vi "Unescape String.vi"(11 "string":string) -> (3 "parsed string":string)   [LabVIEW 2017, in "NI_LVConfig.lvlib"]
uses:
  <vilib>/Utility/config.llb/NI_LVConfig.lvlib
panel:
  out "error out":errorcluster
  in  "error in (no error)":errorcluster
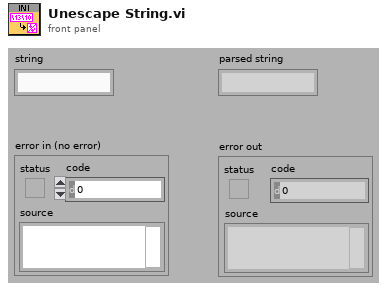
[diagram p1: front panel]
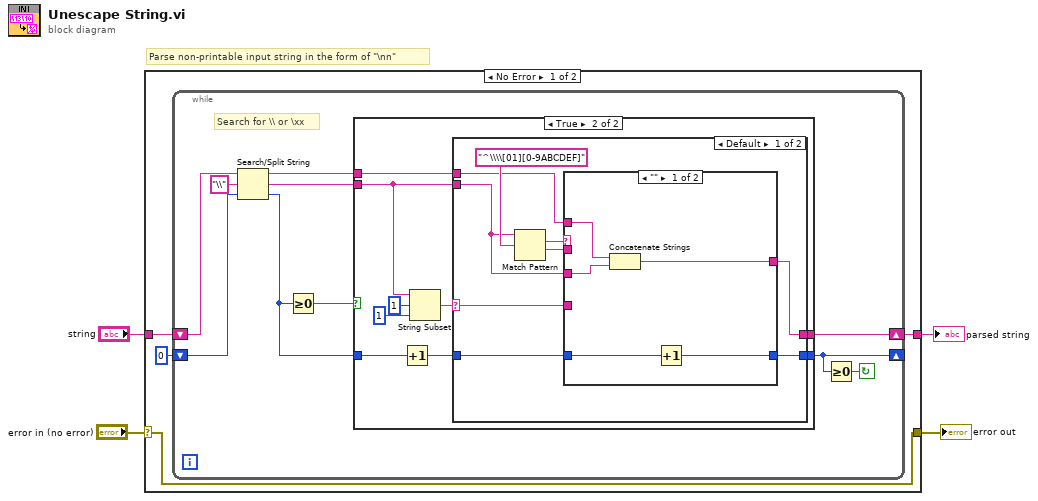
[diagram p0: block diagram]
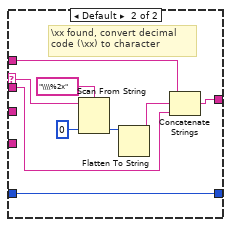
[diagram p3: hidden frame]
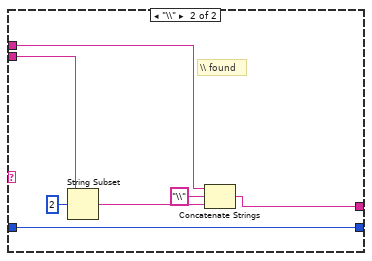
[diagram p4: hidden frame]
diagram:
  # "Parse non-printable input string in the form of \"\\nn\""
  n1 = case shown="No Error" "error in (no error)" {
    selector: "error in (no error)" -> [w5 w60]
    tunnel: "string" -> [w7 w61]
    tunnel: [w6 w61] -> w2
    tunnel: [w5 w60] -> w1
    frame No Error {
      n2 = while {
        shift-left: 0 -> [w14]
        shift-right: [w16] -> _
        shift-left: w7 -> [w15]
        shift-right: [w18] -> w6
        stop <- w17 continue-if-true
        # "Search for \\\\ or \\xx"
        n3 = Search/Split String(string=w15, search string/char (-)="\\", offset (0)=w14) -> (substring before match=w10:string, match + rest of string=w9:string, offset of match=w11:i32)
        n4 = Greater Or Equal To 0?(x=w11) -> (x >= 0?=w12:bool)
        n5 = case shown="True" w12 {
          tunnel: [w20 w29] -> w18
          tunnel: w11 -> [w19 w24]
          tunnel: [w19 w28] -> w16
          tunnel: w10 -> [w20 w27]
          tunnel: w9 -> [_ w23]
          frame False {
          }
          frame True {
            n6 = Increment(x=w24) -> (x+1=w21:i32)
            n7 = String Subset(string=w23, offset (0)=1, length (rest)=1 ("length (rest)")) -> (substring=w26:string)
            n8 = case shown="Default" w26 {
              selector: w26 -> [w38 _]
              tunnel: [w33 w59] -> w29
              tunnel: w21 -> [w31 w53]
              tunnel: [w32 w53] -> w28
              tunnel: w27 -> [w34 w57]
              tunnel: w23 -> [w35 w56]
              frame Default {
                n9 = Match Pattern(string=w35, regular expression="^\\\\[01][0-9ABCDEF]") -> (match substring=w36:string, after substring=w30:string)  [unwired: 1 in, 2 out]
                n10 = case shown="\"\"" w36 {
                  selector: w36 -> [_ w49]
                  tunnel: w38 -> [_ _]
                  tunnel: w35 -> [w42 _]
                  tunnel: w34 -> [w43 w47]
                  tunnel: [w41 w48] -> w33
                  tunnel: [w39 w44] -> w32
                  tunnel: w31 -> [w40 w44]
                  tunnel: w30 -> [_ w45]
                  frame "" {
                    n11 = Concatenate Strings(w43, w42) -> (w41:string)
                    n12 = Increment(x=w40) -> (x+1=w39:i32)
                  }
                  frame Default {
                    # "\\xx found, convert decimal \ncode (\\xx) to character"
                    n13 = Scan From String(format string="\\\\%2x" ("Input String"), input string=w49, default 1=u8 0) -> (output 1=w51:u8)  [unwired: 2 in, 3 out]
                    n14 = Flatten To String(anything=w51) -> (data string=w46:string)  [unwired: 1 in, 4 out]
                    n15 = Concatenate Strings(w47, w46, w45) -> (w48:string)
                  }
                }
              }
              frame "\\" {
                # "\\\\ found"
                n16 = String Subset(string=w56, offset (0)=2) -> (substring=w54:string)  [unwired: 1 in]
                n17 = Concatenate Strings(w57, "\\" ("Input String"), w54) -> (w59:string)
              }
            }
          }
        }
        n18 = Greater Or Equal To 0?(x=w16) -> (x >= 0?=w17:bool)
      }
    }
    frame Error {
    }
  }
  "parsed string" <- w2
  "error out" <- w1
